vi "LOGBOT_EPICS.vi"() -> ()   [LabVIEW 2019]
uses:
  <vilib>/Utility/config.llb/Read Key (String).vi
  <userlib>/caLab/Private/Get_PV-1D.vi
  <vilib>/Utility/config.llb/NI_LVConfig.lvlib
panel:
  out "concatenated string 2":string
  out "Past SEStxt":string
  out "SEStxt Current":string
  out "concatenated string":string
  out "Array":bool[](array[boolean])
  out "Array size":i32
  out "Past PVvalue array":string[](array[string])
  out "PVvalue array":string[](array[string])
  out "PVname array":string[](array[string])
  out "HISTORY:maindir":string="P:\\BL13-0\\BL13-2\\HISTORY\\"
  out "BL132:CONFIG":path=path "S:/INI/BL132.INI"
  out "LOGBOT file":path=path "P:/b_ogasawara/BL13-0/BL13-2/HISTORY/171103.csv"
  out "current time":timestamp
  # "SES:filename"
  # "SPEC:filename"
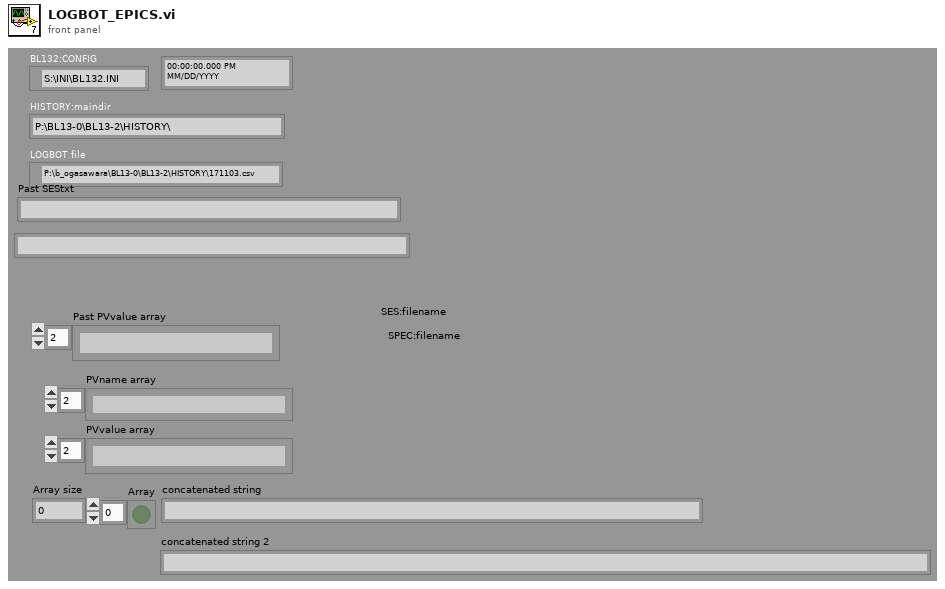
[diagram p1: front panel]
types:
  T1 = typedef "NI_LVConfig.lvlib/Config Data RefNum.ctl" = refnum<k1>
  T2 = enum16{"open", "replace", "create", "open or create", "replace or create", "replace or create with confirmation"}
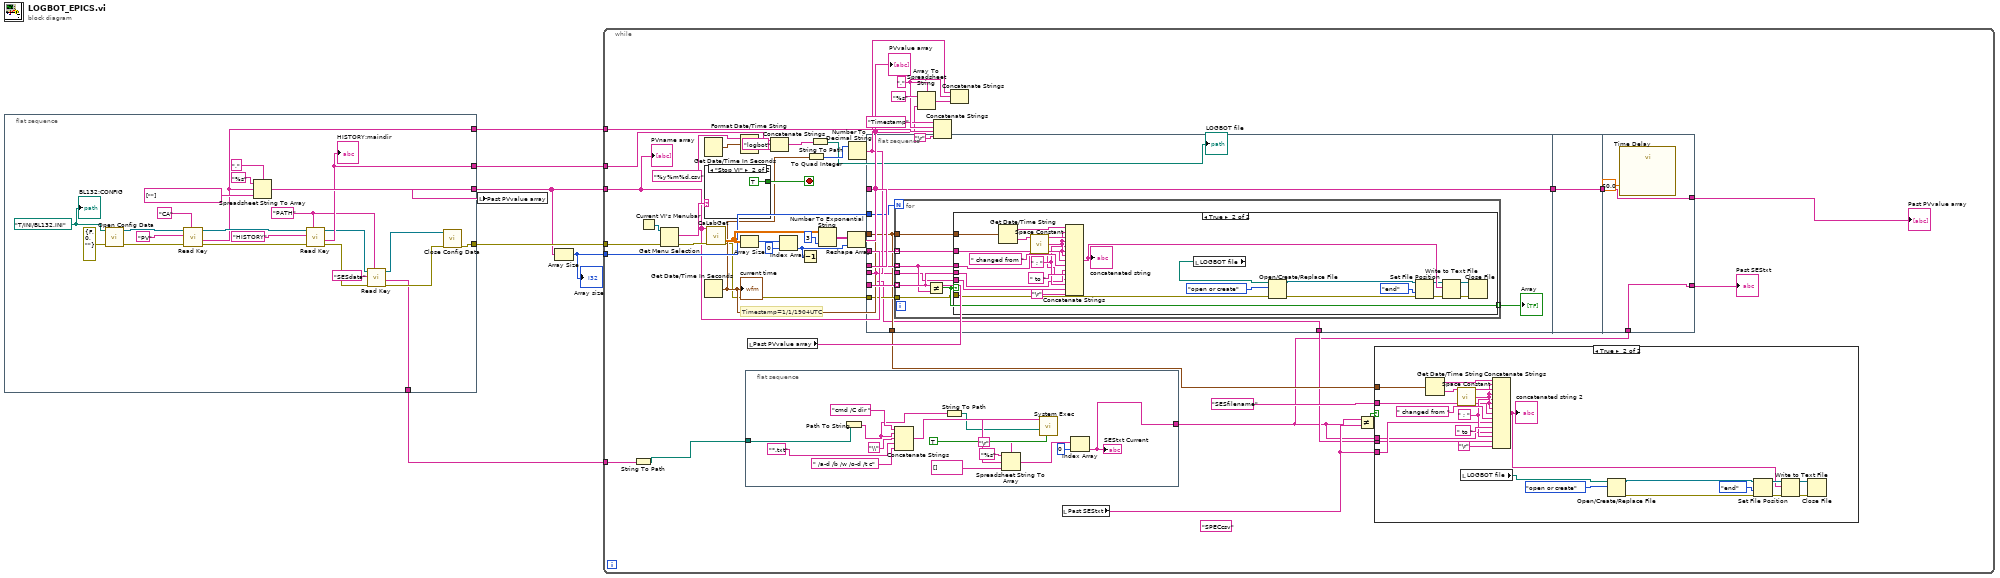
[diagram p0: block diagram]
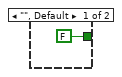
[diagram p4: hidden frame]
diagram:
  n1 = flat-sequence {
    tunnel: [w21] -> w3
    tunnel: [w19] -> w6
    tunnel: [w16] -> w5
    tunnel: [w14] -> w4
    tunnel: [w7] -> w1
    frame #0 {
      w29 = path "T:/INI/BL132.INI" ("configuration file path")
      w11 = "PATH" ("key")
      n2 = call <vilib>:"Open Config Data.vi"("error in (no error)"=errorcluster {"status"=FALSE, "code"=0, "source"=""}, "configuration file path"=w29) -> ("error out"=w17:errorcluster, "refnum"=w26:T1)  [unwired: 7 in, 1 out]
      n3 = call-poly <vilib>:"Read Key.vi"("section"="CA", "error in (no error)"=w17, "key"="PV", "refnum"=w26) -> ("error out"=w18:errorcluster, "value"=w19:string, "refnum out"=w22:T1)  [unwired: 4 in, 1 out]
      n4 = Spreadsheet String To Array(delimiter (Tab)=",", format string="%s", spreadsheet string=w19, array type (2D Dbl)=string[] [""] ("Strings []")) -> (array=w21:string[])
      n5 = call-poly <vilib>:"Read Key.vi"("section"=w11, "error in (no error)"=w18, "key"="HISTORY" ("section"), "refnum"=w22) -> ("error out"=w12:errorcluster, "value"=w14:string, "refnum out"=w13:T1)  [unwired: 4 in, 1 out]
      "HISTORY:maindir" <- w14
      n6 = call-poly <vilib>:"Read Key.vi"("section"=w11, "error in (no error)"=w12, "key"="SESdata", "refnum"=w13) -> ("error out"=w8:errorcluster, "value"=w7:string, "refnum out"=w9:T1)  [unwired: 4 in, 1 out]
      n7 = call <vilib>:"Close Config Data.vi"("error in (no error)"=w8, "refnum"=w9) -> ("error out"=w16:errorcluster)  [unwired: 8 in, 1 out]
      "BL132:CONFIG" <- w29
    }
  }
  n8 = local write "Past PVvalue array"(w3) -> ()
  n9 = Array Size(array=w3) -> (size(s)=w2:i32)
  "Array size" <- w2
  n10 = while {
    tunnel: w3 -> [w45]
    tunnel: w6 -> [w61]
    tunnel: w5 -> [w56]
    tunnel: w4 -> [w53]
    tunnel: w2 -> [w52]
    tunnel: w1 -> [w37]
    stop <- w71 stop-if-true
    (unwired) "SPECcsv" ("HSnap_Filter jpg")
    w63 = "," ("string")
    # "Timestamp=1/1/1904UTC"
    n11 = String To Path(string=w37) -> (path=w38:path)
    n12 = Current VI's Menubar() -> (w73:refnum<k9>)
    n13 = Get Menu Selection(0:w73, 3:w56) -> (6:w72:string, 8:w55:errorcluster)  [unwired: 2 in, 3 out]
    n14 = Get Date/Time In Seconds() -> (seconds since 1Jan1904=w64:timestamp)
    n15 = case shown="\"Stop VI\"" w72 {
      tunnel: [FALSE TRUE] -> w71
      frame "", Default {
      }
      frame "Stop VI" {
      }
    }
    n16 = Get Date/Time In Seconds() -> (seconds since 1Jan1904=w43:timestamp)
    "current time" <- w43
    n17 = call-poly <userlib>:"CaLabGet.vi"("PV Names"=w45, "Error in (no error)"=w55) -> ("Value Array (number)"=w59:dbl[][], "Error out"=w42:errorcluster)  [unwired: 7 in, 5 out]
    n18 = Format Date/Time String(time format string (%c)="%y%m%d.csv", seconds (now)=w64) -> (date/time string=w41:string)  [unwired: 1 in]
    n19 = Array Size(array=w59) -> (size(s)=w58:i32[])
    n20 = flat-sequence {
      tunnel: w38 -> [w105]
      tunnel: [w96] -> w31
      frame #0 {
        n21 = Path To String(path=w105) -> (string=w97:string)
        n22 = Concatenate Strings("cmd /C dir " ("command line"), w97, "\\" ("string"), "*.txt" ("HSnap_Filter jpg"), " /a-d /b /w /o-d /t c" ("command line")) -> (w106:string)
        n23 = String To Path(string=w97) -> (path=w100:path)
        n24 = call <vilib>:"System Exec.vi"("run minimized? (F)"=TRUE, "working directory"=w100, "command line"=w106) -> ("standard output"=w110:string)  [unwired: 3 in, 5 out]
        n25 = Spreadsheet String To Array(delimiter (Tab)="\r", format string="%s", spreadsheet string=w110, array type (2D Dbl)=string[] []) -> (array=w104:string[])
        n26 = Index Array(array=w104, index=0) -> (element=w96:string)
        "SEStxt Current" <- w96
      }
    }
    n27 = local read "Past PVvalue array"() -> (w49:string[])
    n28 = Concatenate Strings(w53, "logbot" ("string"), w41) -> (w66:string)
    n29 = Index Array(array=w58, index=0 ("dimension size")) -> (element=w54:i32)
    n30 = Decrement(x=w54) -> ()  [unwired: 1 out]
    n31 = To Quad Integer(1:w43) -> (0:w67:i64)
    n32 = String To Path(string=w66) -> (path=→"LOGBOT file":path)
    n33 = Number To Exponential String(number=w59, precision (6)=i16 3) -> (E-format string=w70:string[][])  [unwired: 2 in]
    n34 = Reshape Array(w70, w54) -> (w51:string[])
    "PVvalue array" <- w51
    n35 = Number To Decimal String(number=w67) -> (decimal integer string=w44:string)  [unwired: 1 in]
    n36 = flat-sequence {
      tunnel: w52 -> [w120]
      tunnel: w51 -> [w119]
      tunnel: w49 -> [w118]
      tunnel: w51 -> [w116]
      tunnel: [w116] -> w47
      tunnel: w45 -> [w115]
      tunnel: w44 -> [w112]
      tunnel: w43 -> [w113]
      tunnel: w42 -> [w114]
      tunnel: [w113] -> w35
      tunnel: [w112] -> w32
      tunnel: w47 -> [w151]
      tunnel: [w151] -> w46
      tunnel: [w154] -> w50
      tunnel: w46 -> [w154]
      tunnel: [w152] -> w36
      tunnel: w31 -> [w152]
      frame #0 {
        n37 = for {
          N: w120 -> [_]
          tunnel: w119 -> [w125] mode=indexing
          tunnel: w118 -> [w124] mode=indexing
          tunnel: [w127] -> w117 mode=indexing
          tunnel: w115 -> [w126] mode=indexing
          tunnel: w112 -> [w123]
          tunnel: w113 -> [w122]
          tunnel: w114 -> [w121]
          n38 = Not Equal?(x=w124, y=w125) -> (x != y?=w127:bool)
          n39 = case shown="True" w127 {
            tunnel: w126 -> [_ w149]
            tunnel: w125 -> [_ w128]
            tunnel: w124 -> [_ w129]
            tunnel: w123 -> [_ w139]
            tunnel: w122 -> [_ w147]
            tunnel: w121 -> [_ w142]
            frame False {
            }
            frame True {
              w143 = " ; " ("string")
              n40 = Get Date/Time String(seconds (now)=w147) -> (date string=w146:string, time string=w145:string)  [unwired: 2 in]
              n41 = call <vilib>:"Space Constant.vi"() -> ("String"=w144:string)
              n42 = Concatenate Strings(w146, w144, w145, w144, w143, w144, w144, w149, " changed from ", w129, " to ", w128, w143, w139, "\r") -> (w141:string)
              "concatenated string" <- w141
              n43 = local read "LOGBOT file"() -> (w132:path)
              n44 = Open/Create/Replace File(file path (use dialog)=w132, error in=w142, operation (0:open)=T2."open or create" ("operation (0:open) 2")) -> (refnum out=w131:refnum<file>, error out=w130:errorcluster)  [unwired: 3 in, 1 out]
              n45 = Set File Position(refnum=w131, from (0:start)=enum16{"start", "end", "current"}."end", error in=w130) -> (refnum out=w136:refnum<file>, error out=w134:errorcluster)  [unwired: 1 in]
              n46 = Write to Text File(file (use dialog)=w136, text=w141, error in=w134) -> (refnum out=w138:refnum<file>, error out=w133:errorcluster)  [unwired: 1 in, 1 out]
              n47 = Close File(refnum=w138, error in=w133) -> ()  [unwired: 2 out]
            }
          }
        }
        "Array" <- w117
      }
      frame #1 {
      }
      frame #2 {
        n48 = call "Time Delay"("Delay Time (s)"=60.0) -> ()  [unwired: 10 in, 1 out]
      }
    }
    n49 = Array To Spreadsheet String(delimiter (Tab)=w63, array=w51, 3:"%s" ("format string")) -> (spreadsheet string=w68:string)
    n50 = Concatenate Strings("Timestamp" ("format string"), w63, w61, "\r") -> ()  [unwired: 1 out]
    n51 = Concatenate Strings(w44, w63, w68) -> ()  [unwired: 1 out]
    n52 = local read "Past SEStxt"() -> (w34:string)
    n53 = Not Equal?(x=w31, y=w34) -> (x != y?=w30:bool)
    n54 = case shown="True" w30 {
      tunnel: w35 -> [_ w88]
      tunnel: w34 -> [_ w87]
      tunnel: "SESfilename" -> [_ w86]
      tunnel: w32 -> [_ w85]
      tunnel: w31 -> [_ w84]
      frame False {
      }
      frame True {
        w90 = " ; " ("string")
        n55 = Get Date/Time String(seconds (now)=w88) -> (date string=w93:string, time string=w92:string)  [unwired: 2 in]
        n56 = call <vilib>:"Space Constant.vi"() -> ("String"=w91:string)
        n57 = local read "LOGBOT file"() -> (w75:path)
        n58 = Concatenate Strings(w93, w91, w92, w91, w90, w91, w91, w86, " changed from ", w87, " to ", w84, w90, w85, "\r") -> (w74:string)
        "concatenated string 2" <- w74
        n59 = Open/Create/Replace File(file path (use dialog)=w75, operation (0:open)=T2."open or create" ("operation (0:open) 2")) -> (refnum out=w77:refnum<file>, error out=w76:errorcluster)  [unwired: 4 in, 1 out]
        n60 = Set File Position(refnum=w77, from (0:start)=enum16{"start", "end", "current"}."end", error in=w76) -> (refnum out=w81:refnum<file>, error out=w79:errorcluster)  [unwired: 1 in]
        n61 = Write to Text File(file (use dialog)=w81, text=w74, error in=w79) -> (refnum out=w83:refnum<file>, error out=w78:errorcluster)  [unwired: 1 in, 1 out]
        n62 = Close File(refnum=w83, error in=w78) -> ()  [unwired: 2 out]
      }
    }
    "PVname array" <- w45
    "Past PVvalue array" <- w50
    "Past SEStxt" <- w36
  }
